vi "Indexing maapped image indicator array.vi"(8 "Rack Id":u8, 9 "Image update":cluster{"Rack Id":i32, "Update image":bool[]}[](array[cluster])=[{"Rack Id"=0, "Update image"=[TRUE, TRUE, FALSE, FALSE]}, {"Rack Id"=1, "Update image"=[FALSE, FALSE, TRUE, TRUE]}], 10 "ISIM":u8[](array[numeric]), 11 "Image array":T1[](array[typedef])) -> (1 "Table update":bool[](array[boolean]), 2 "Update image":bool[](array[boolean]), 3 "mapped image arr out":T1[](array[typedef]))   [LabVIEW 2019, in "ZenGage v3.0 UI.lvclass"]
uses:
  ZenGage v3.0 UI.lvclass
  <vilib>/vision/Image Controls.llb/IMAQ Image.ctl
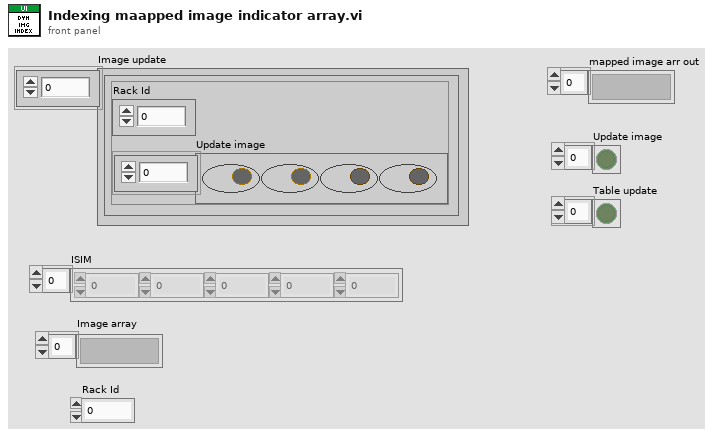
[diagram p1: front panel]
types:
  T1 = typedef "IMAQ Image.ctl" = refnum<image>
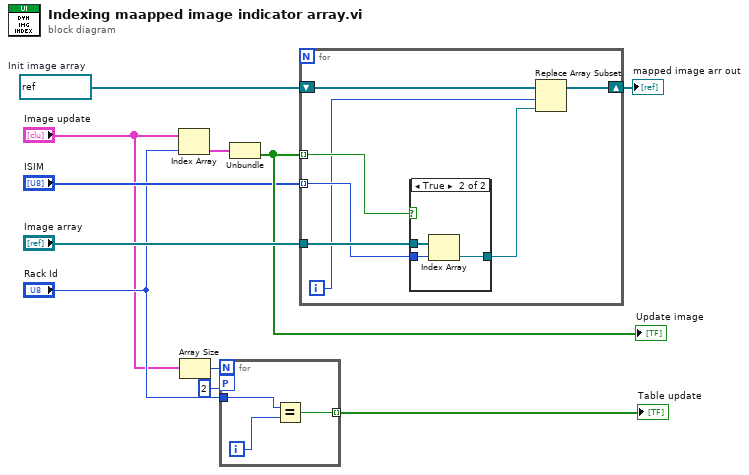
[diagram p0: block diagram]
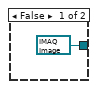
[diagram p2: hidden frame]
diagram:
  w8 = T1[] ["test 1", "test 2", "test 3", "test 4"]  # Init image array
  n1 = Index Array(array="Image update", index="Rack Id") -> (element=w11:cluster{"Rack Id":i32, "Update image":bool[]})
  n2 = Array Size(array="Image update") -> (size(s)=w3:i32)
  n3 = for {
    N: w3 -> [_]
    tunnel: "Rack Id" -> [w14]
    tunnel: [w12] -> w2 mode=indexing
    workers-P: 2 -> [_]
    i -> [w13]
    n4 = Equal?(x=w14, y=w13) -> (x = y?=w12:bool)
  }
  "Table update" <- w2
  n5 = Unbundle(w11) -> ("Update image"=w9:bool[])  [unwired: 1 out]
  "Update image" <- w9
  n6 = for {
    tunnel: "Image array" -> [w21]
    tunnel: w9 -> [w20] mode=indexing
    tunnel: "ISIM" -> [w19] mode=indexing
    shift-right: [w15] -> w6
    shift-left: w8 -> [w18]
    i -> [w16]
    n7 = case shown="True" w20 {
      tunnel: w21 -> [_ w25]
      tunnel: w19 -> [_ w24]
      tunnel: [T1 refnum ("Image") w23] -> w17
      frame False {
      }
      frame True {
        n8 = Index Array(array=w25, index=w24) -> (element=w23:T1)
      }
    }
    n9 = Replace Array Subset(array=w18, new element=w17, index=w16) -> (w15:T1[])
  }
  "mapped image arr out" <- w6
